vi "FeedForward_src.vi"(7 "wL_factor":sgl=0.11000061, 8 "FeedForwardEnable":bool, 9 "GridIdq":T1, 10 "GridVdq":T1={"D"=216.45131, "Q"=0.0}, 11 "Vcmd":T1) -> (3 "VcmdWithFeedForward":T1)   [LabVIEW 2015]
uses:
  AFE/DQ.ctl
  AFE/ActiveFrontEnd.lvlib
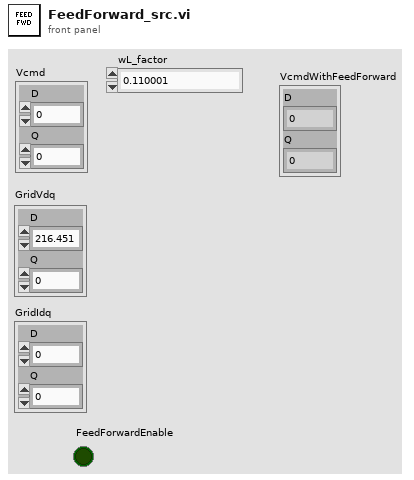
[diagram p1: front panel]
types:
  T1 = typedef "ActiveFrontEnd.lvlib/DQ.ctl" = cluster{"D":sgl, "Q":sgl}
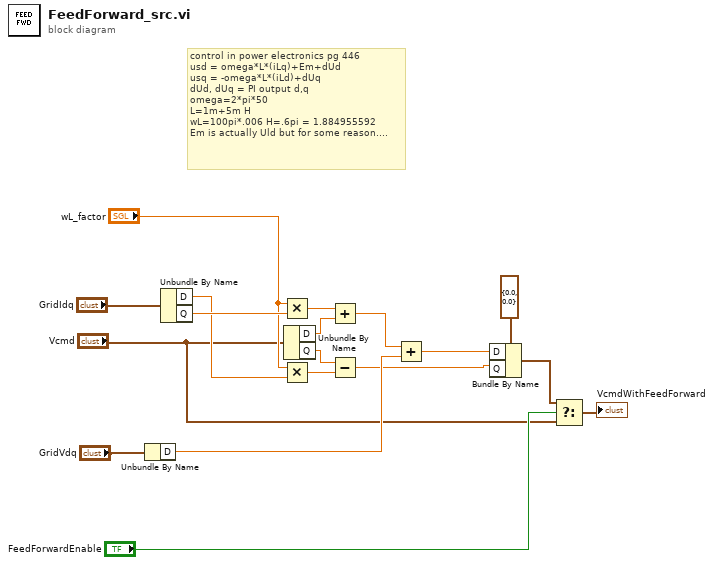
[diagram p0: block diagram]
diagram:
  # "control in power electronics pg 446\nusd = omega*L*(iLq)+Em+dUd\nusq = -omega*L*(iLd)+dUq\ndUd, dUq = PI output d,q\nomega=2*pi*50\nL=1m+5m H\nwL=100pi*.006 H=.6pi = 1.884955592\nEm is actually Uld but for some reason...."
  n1 = Unbundle By Name("GridVdq") -> ("D"=w8:sgl)
  n2 = Unbundle By Name("GridIdq") -> ("D"=w13:sgl, "Q"=w18:sgl)
  n3 = Multiply(x="wL_factor", y=w18) -> (x*y=w17:sgl)
  n4 = Multiply(x="wL_factor", y=w13) -> (x*y=w11:sgl)
  n5 = Unbundle By Name("Vcmd") -> ("D"=w15:sgl, "Q"=w14:sgl)
  n6 = Add(x=w17, y=w15) -> (x+y=w16:sgl)
  n7 = Subtract(x=w14, y=w11) -> (x-y=w5:sgl)
  n8 = Add(x=w16, y=w8) -> (x+y=w6:sgl)
  n9 = Bundle By Name(cluster=T1 {"D"=0.0, "Q"=0.0} ("Vcmd"), "D"=w6, "Q"=w5) -> (w3:T1)
  n10 = Select(t=w3, s="FeedForwardEnable", f="Vcmd") -> (s? t:f=→"VcmdWithFeedForward":T1)
